vi "Init - Copia.vi"(8 "error in (no error)":errorcluster, 10 "ICameraTestingUI":refnum<class "ICameraTestingUI.lvclass">, 11 "CameraTesting in":refnum<class "CameraTesting.lvclass">) -> (0 "error out":errorcluster, 3 "CameraTesting out":refnum<class "CameraTesting.lvclass">)   [LabVIEW 2020, in "CameraTesting.lvlib" / "CameraTesting.lvclass"]
uses:
  CameraTesting.lvclass
  C:/Program Files (x86)/National Instruments/LabVIEW 2020/vi.lib/ActorFramework/Actor/Actor.lvclass
  ICameraTestingUI/ICameraTestingUI/ICameraTestingUI.lvclass
  <vilib>/ActorFramework/Actor/Actor.lvclass
  CameraTesting.lvclass/CameraTesting.ctl
  Private/TypeDef/MsgInitStates.ctl
  Camera/ICamera/ICamera/ICamera.lvclass
  E:/GitHub/Evaluation_Test/Labview/src/CameraTestingApp/CameraTesting/CameraTesting/CameraTesting.lvclass
  E:/GitHub/Evaluation_Test/Labview/src/CameraTestingApp/ICameraTesting/ICameraTesting/ICameraTesting.lvclass
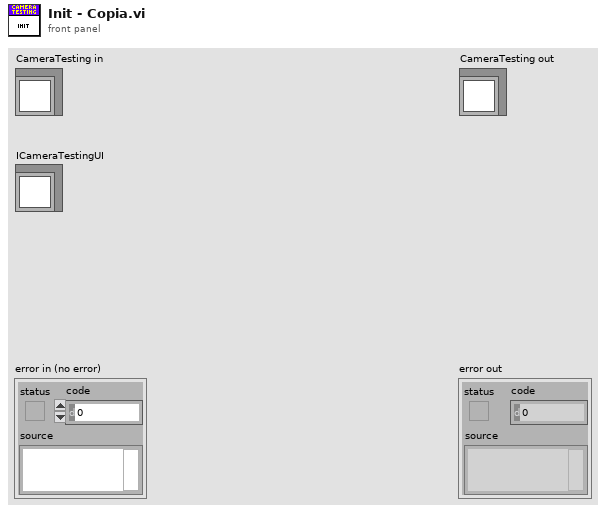
[diagram p1: front panel]
types:
  T1 = typedef "CameraTesting.lvlib/CameraTesting.lvclass/MsgInitStates.ctl" = enum16{"Inizialize Camera", "Camera Events Request", "Enumeration Camera Video Options", "Events Registration", "Launch User Interface", "Show UI"}
  T2 = typedef "ICamera.lvlib/ICamera.lvclass/Events.ctl" = cluster{"CameraStreamDataUpdate":T3}
  T3 = typedef "ICamera.lvlib/ICamera.lvclass/StreamDataEvent.ctl" = refnum<user-event>
  T4 = typedef "ICamera.lvlib/ICamera.lvclass/VideoOptionsCodes.ctl" = cluster{"FrameRateCodesList":cluster{"Description":string, "Code":u8}[], "VideoResolutionCodesList":cluster{"Description":string, "Code":u8}[], "ImageTypeCodesList":cluster{"Description":string, "Code":u8}[]}
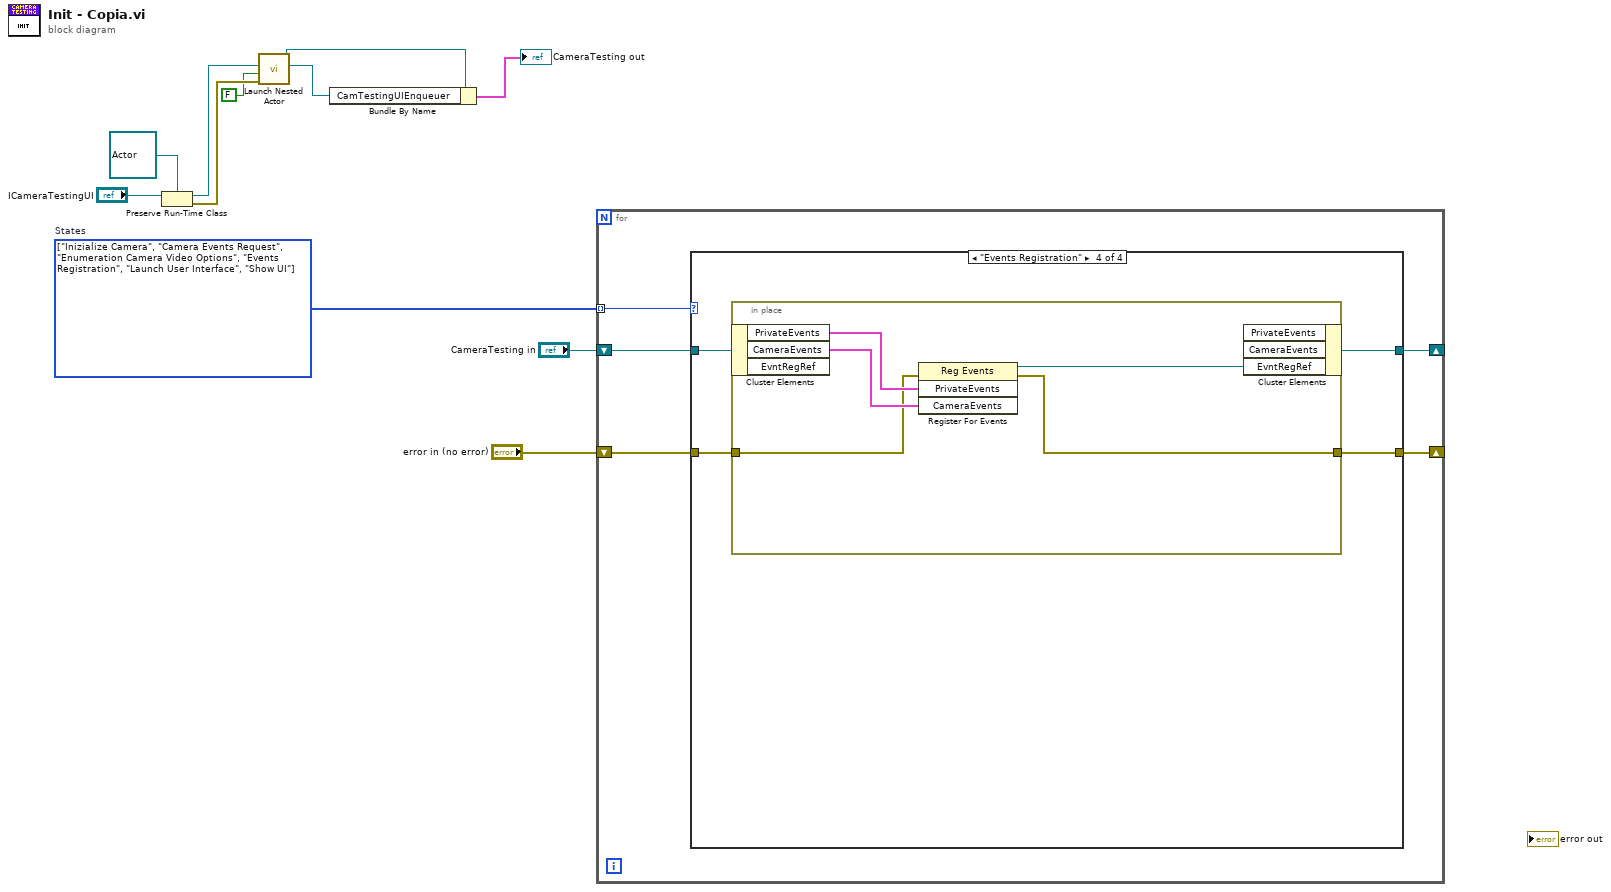
[diagram p0: block diagram]
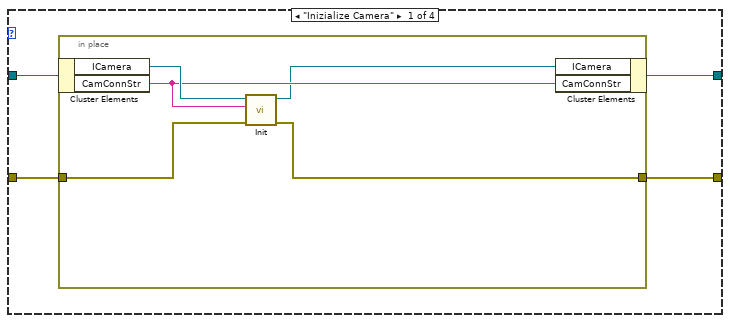
[diagram p2: hidden frame]
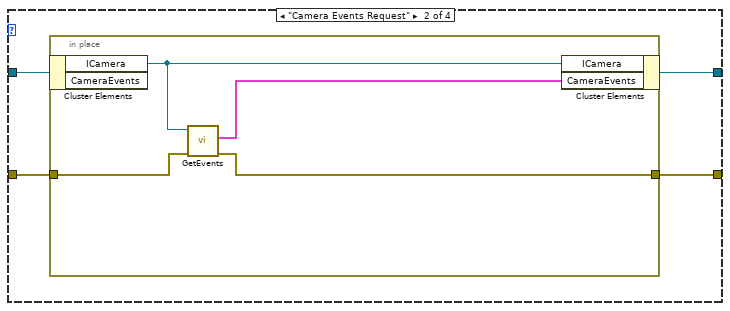
[diagram p3: hidden frame]
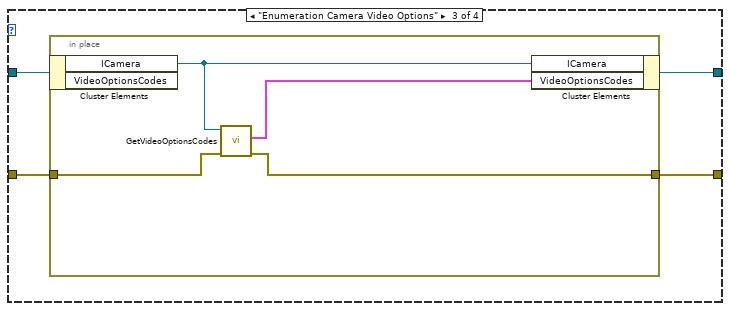
[diagram p4: hidden frame]
diagram:
  w3 = T1[] [enum."Inizialize Camera", enum."Camera Events Request", enum."Enumeration Camera Video Options", enum."Events Registration", enum."Launch User Interface", enum."Show UI"] items=["Inizialize Camera", "Camera Events Request", "Enumeration Camera Video Options", "Events Registration", "Launch User Interface", "Show UI"]  # States
  n1 = Preserve Run-Time Class(object in="ICameraTestingUI", 2:refnum<class "Actor.lvclass"> refnum ("Caller Actor in")) -> (object out=w9:refnum<class "Actor.lvclass">, error out=w8:errorcluster)  [unwired: 1 in]
  n2 = call <vilib>:"Launch Nested Actor.vi"("error in (no error)"=w8, "Auto-stop? (T)"=FALSE, "Nested Actor"=w9) -> ("Nested Actor's Enqueuer"=w5:refnum<class "Message Enqueuer.lvclass">, "Caller Actor out"=w7:refnum<class "Actor.lvclass">)  [unwired: 6 in, 1 out]
  n3 = Bundle By Name(cluster=w7, "CamTestingUIEnqueuer"=w5) -> (→"CameraTesting out":cluster{})
  n4 = for {
    tunnel: w3 -> [w16] mode=indexing
    shift-right: [w12] -> _
    shift-left: "CameraTesting in" -> [w15]
    shift-right: [w13] -> _
    shift-left: "error in (no error)" -> [w14]
    n5 = case shown="\"Events Registration\"" w16 {
      tunnel: w15 -> [w20 w29 w37 w45]
      tunnel: w14 -> [w19 w28 w36 w44]
      tunnel: [w18 w27 w35 w43] -> w13
      tunnel: [w17 w26 w34 w42] -> w12
      frame "Inizialize Camera" {
        n6 = in-place {
          in-place-border: w19 -> [w22]
          in-place-border: [w21] -> w18
          n7 = in-place-cluster #1(w20) -> ("ICamera"=w25:refnum<class "ICamera.lvclass">, "CamConnStr"=w24:string)
          n8 = call-dynamic "Init.vi"("error in (no error)"=w22, "Connection String"=w24, "ICamera in"=w25) -> ("error out"=w21:errorcluster, "ICamera out"=w23:refnum<class "ICamera.lvclass">)  [unwired: 7 in]
          n9 = in-place-cluster #1("ICamera"=w23, "CamConnStr"=w24) -> (w17:refnum<class "CameraTesting.lvclass">)
        }
      }
      frame "Camera Events Request" {
        n10 = in-place {
          in-place-border: w28 -> [w31]
          in-place-border: [w30] -> w27
          n11 = in-place-cluster #2(w29) -> ("ICamera"=w33:refnum<class "ICamera.lvclass">)  [unwired: 1 out]
          n12 = call-dynamic "GetEvents.vi"("error in (no error)"=w31, "ICamera in"=w33) -> ("error out"=w30:errorcluster, "CameraEvents"=w32:T2)  [unwired: 7 in, 1 out]
          n13 = in-place-cluster #2("ICamera"=w33, "CameraEvents"=w32) -> (w26:refnum<class "CameraTesting.lvclass">)
        }
      }
      frame "Enumeration Camera Video Options" {
        n14 = in-place {
          in-place-border: w36 -> [w41]
          in-place-border: [w40] -> w35
          n15 = in-place-cluster #3(w37) -> ("ICamera"=w39:refnum<class "ICamera.lvclass">)  [unwired: 1 out]
          n16 = call-dynamic "GetVideoOptionsCodes.vi"("error in (no error)"=w41, "ICamera in"=w39) -> ("error out"=w40:errorcluster, "VideoOptionsCodes"=w38:T4)  [unwired: 7 in, 1 out]
          n17 = in-place-cluster #3("ICamera"=w39, "VideoOptionsCodes"=w38) -> (w34:refnum<class "CameraTesting.lvclass">)
        }
      }
      frame "Events Registration" {
        n18 = in-place {
          in-place-border: w44 -> [w47]
          in-place-border: [w46] -> w43
          n19 = in-place-cluster #4(w45) -> ("PrivateEvents"=w50:cluster{"ActorStopped":refnum<user-event>}, "CameraEvents"=w49:T2)  [unwired: 1 out]
          n20 = register-events(error in=w47, w50, w49) -> (reference out=w48:refnum<event-registration>, error out=w46:errorcluster)  [unwired: 1 in]
          n21 = in-place-cluster #4("EvntRegRef"=w48) -> (w42:refnum<class "CameraTesting.lvclass">)  [unwired: 2 in]
        }
      }
    }
  }
